vi "SV TDMS Write Waveform (1 Ch).vi"(0 "tdms file":refnum<k34>, 1 "write channel properties (T)":bool=TRUE, 5 "group name in":string="Waveform", 7 "channel name in":string="Channel0", 9 "scaled signal [EU]":waveform(dbl), 11 "error in":errorcluster) -> (4 "tdms file out":refnum<k34>, 6 "group name out":string, 8 "channel name out":string, 15 "error out":errorcluster)   [LabVIEW 2017]
doc: "Writes data to the specified .tdms file in a format specific to the polymorphic instance. Wire data to the <B>scaled signal [EU]</B> input to determine the polymorphic instance to use or manually select the instance."
uses:
  <vilib>/addons/_NISVFA/_Shared subVIs/Controls/LV Datatypes.ctl
  <vilib>/addons/_NISVFA/_Shared subVIs/Controls/NI Function Info.ctl
  <vilib>/addons/_NISVFA/_Shared subVIs/Controls/NI Function Type.ctl
  <vilib>/addons/_NISVFA/_Shared subVIs/Controls/NI Function SubType.ctl
  <vilib>/addons/_NISVFA/_Shared subVIs/Controls/svc_X-Axis Units.ctl
  <vilib>/addons/_NISVFA/_Shared subVIs/Controls/svc_Unit Info.ctl
  <vilib>/addons/_NISVFA/_Shared subVIs/Common/svc_Engineering Units to Unit Label.vi
  <vilib>/addons/_NISVFA/_Shared subVIs/Common/svc_Unit Label to Engineering Units.vi
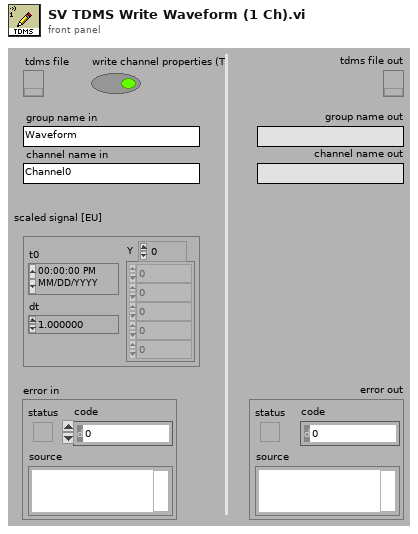
[diagram p1: front panel]
types:
  T1 = typedef "svc_Unit Info.ctl" = cluster{"X-axis label":string, "X-unit string":string, "Y-axis label":string, "Y-unit string":string}
  T2 = typedef "NI Function Info.ctl" = cluster{"function type":T3, "function subtype":T4, "X-dimension":T5}
  T3 = typedef "NI Function Type.ctl" = u16
  T4 = typedef "NI Function SubType.ctl" = u16
  T5 = typedef "svc_X-Axis Units.ctl" = u16
  T6 = typedef "LV Datatypes.ctl" = i32
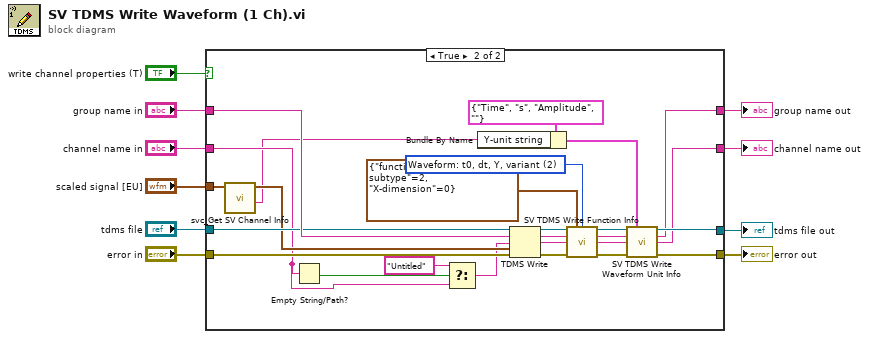
[diagram p0: block diagram]
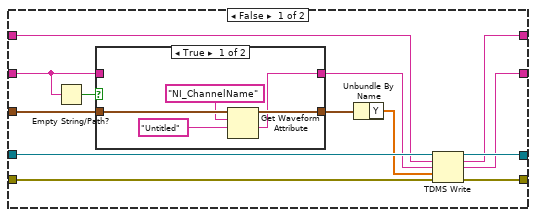
[diagram p2: hidden frame]
diagram:
  n1 = case shown="True" "write channel properties (T)" {
    tunnel: [w18 w47] -> w10
    tunnel: [w13 w42] -> w9
    tunnel: "channel name in" -> [w23 w36]
    tunnel: "group name in" -> [w11 w56]
    tunnel: "tdms file" -> [w19 w55]
    tunnel: "scaled signal [EU]" -> [w21 w54]
    tunnel: [w17 w40] -> w4
    tunnel: [w16 w41] -> w3
    tunnel: "error in" -> [w12 w52]
    frame False {
      n2 = Empty String/Path?(string/path=w23) -> (empty?=w22:bool)
      n3 = case shown="True" w22 {
        tunnel: w23 -> [_ w29]
        tunnel: w21 -> [w28 w30]
        tunnel: [w27 w30] -> w20
        tunnel: [w24 w29] -> w14
        frame True {
          n4 = Get Waveform Attribute(5:"Untitled" ("t"), 6:"NI_ChannelName" ("name"), 7:w28) -> (1:w24:string, 3:w27:waveform(dbl))  [unwired: 1 in, 2 out]
        }
        frame False {
        }
      }
      n5 = Unbundle By Name(w20) -> ("Y"=w15:dbl[])
      n6 = TDMS Write(0:w19, 5:w11, 7:w14, 9:w15, 11:w12) -> (4:w18:refnum<k34>, 6:w17:string, 8:w16:string, 15:w13:errorcluster)  [unwired: 1 in]
    }
    frame True {
      w38 = T6 2 items=["String"=-2, "Boolean"=-1, "Scalar: y"=0, "Array: Y"=1, "Waveform: t0, dt, Y, variant"=2, "Cluster: x0, dx, Y"=3, "Cluster: X, Y"=4, "Waterfall"=5, "Colormap"=6] ("LabVIEW datatype")
      n7 = call <vilib>:"svc_Get SV Channel Info.vi"("scaled signal [EU]"=w54) -> ("unit label"=w32:string, "dup scaled signal [EU]"=w53:waveform(dbl))  [unwired: 5 in, 4 out]
      n8 = Empty String/Path?(string/path=w36) -> (empty?=w37:bool)
      n9 = Select(t="Untitled", s=w37, f=w36) -> (s? t:f=w35:string)
      n10 = Bundle By Name(cluster=T1 {"X-axis label"="Time", "X-unit string"="s", "Y-axis label"="Amplitude", "Y-unit string"=""} ("unit info"), "Y-unit string"=w32) -> (w31:T1)
      n11 = TDMS Write(0:w55, 5:w56, 7:w35, 9:w53, 11:w52) -> (4:w46:refnum<k34>, 6:w45:string, 8:w44:string, 15:w43:errorcluster)  [unwired: 1 in]
      n12 = call <vilib>:"SV TDMS Write Function Info.vi"("tdms file in"=w46, "function info"=T2 {"function type"=0, "function subtype"=2, "X-dimension"=0}, "LabVIEW datatype"=w38, "group name"=w45, "channel name"=w44, "error in (no error)"=w43) -> ("tdms file out"=w51:refnum<k34>, "group name out"=w50:string, "channel name out"=w49:string, "error out"=w48:errorcluster)  [unwired: 6 in]
      n13 = call <vilib>:"SV TDMS Write Waveform Unit Info.vi"("tdms file"=w51, "unit info"=w31, "group name"=w50, "channel name"=w49, "error in (no error)"=w48) -> ("tdms file out"=w47:refnum<k34>, "group name out"=w40:string, "channel name out"=w41:string, "error out"=w42:errorcluster)  [unwired: 7 in]
    }
  }
  "tdms file out" <- w10
  "error out" <- w9
  "channel name out" <- w3
  "group name out" <- w4
